vi "Get Datatype.vi"(8 "error in (no error)":errorcluster, 11 "Object in":refnum<class "Object.lvclass">) -> (0 "error out":errorcluster, 2 "Datatype":T1, 3 "Object out":refnum<class "Object.lvclass">)   [LabVIEW 2019, in "HierDAL Library.lvlib" / "Models.lvlib" / "Object.lvclass"]
uses:
  Object.lvclass
  Common Library/Controls/Datatype.ctl
  Object.lvclass/Object.ctl
  Common Library/Common.lvlib
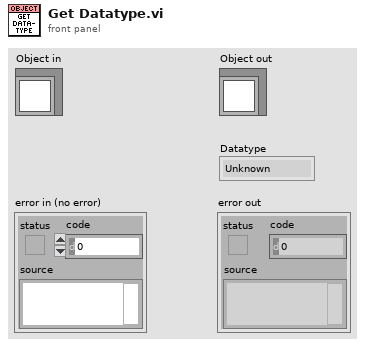
[diagram p1: front panel]
types:
  T1 = typedef "HierDAL Library.lvlib/Common.lvlib/Datatype.ctl" = enum16{"Unknown", "Group", "Dataset"}
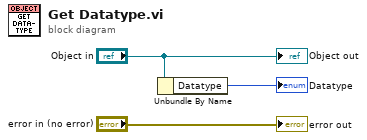
[diagram p0: block diagram]
diagram:
  n1 = Unbundle By Name("Object in") -> ("Datatype"=→"Datatype":T1)
  "error out" <- "error in (no error)"
  "Object out" <- "Object in"
